vi "busy_wait.vi"(7 "caller":refnum<vi>, 8 "error in (no error)":errorcluster, 10 "configuration":T2={"dialog_text"="", "wait_s"=0.0, "inner_color"=16711680, "outer_color"=6618880, "event_registration"=refnum}, 11 "v1 in":refnum<class "v1.lvclass">) -> (0 "error out":errorcluster, 2 "dialog_selection":T1, 3 "v1 out":refnum<class "v1.lvclass">)   [LabVIEW 2015, in "lv-dialog.lvlib" / "v1.lvlib" / "v1.lvclass"]
doc: "The busy/wait api can be used to provide feedback when a process is going to take a long time, as implemented within the base api class, it doesn't have a lot of functional feedback aside from setting or unsetting busy. The configuration provides a time (in seconds), the dialog message as well as an event registration that can be used to indicate \"done\" from the outside.\n\nThis is implemented by the base api class (not the embedded) by using the \"Set Busy\" and \"Unset Busy\" VIs."
uses:
  v1.lvclass
  _controls/selection.ctl
  v1.lvlib
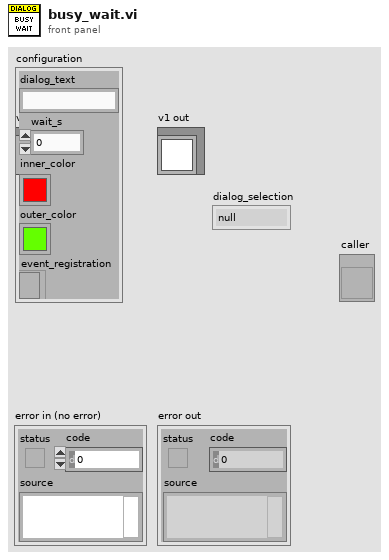
[diagram p1: front panel]
types:
  T1 = typedef "lv-dialog.lvlib/v1.lvlib/selection.ctl" = enum16{"null", "panel_closed", "button_1", "button_2", "button_3", "cancelled"}
  T2 = cluster{"dialog_text":string, "wait_s":dbl, "inner_color":u32, "outer_color":u32, "event_registration":refnum<event-registration>}
  T3 = cluster{"dialog_text":string, "boolean_text_1":string, "boolean_text_2":string}
  T4 = cluster{"dialog_text":string, "boolean_text_1":string}
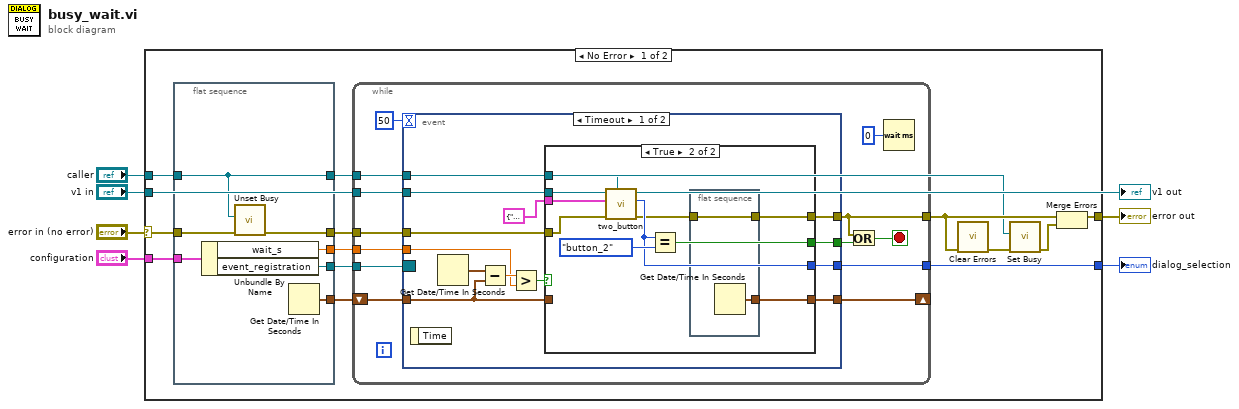
[diagram p0: block diagram]
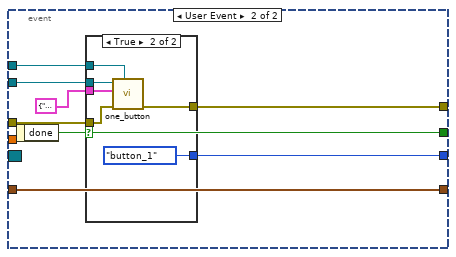
[diagram p3: hidden frame]
diagram:
  n1 = case shown="No Error" "error in (no error)" {
    selector: "error in (no error)" -> [w14 w83]
    tunnel: "configuration" -> [w20 _]
    tunnel: [w17 _] -> w5
    tunnel: "v1 in" -> [w16 _]
    tunnel: "caller" -> [w13 _]
    tunnel: [w9 w83] -> w1
    frame No Error {
      n2 = flat-sequence {
        tunnel: w20 -> [w27]
        tunnel: [w26] -> w19
        tunnel: [w25] -> w18
        tunnel: [w24] -> w15
        tunnel: w14 -> [w23]
        tunnel: w13 -> [w22]
        tunnel: [w22] -> w7
        tunnel: [w21] -> w12
        frame #0 {
          n3 = Unbundle By Name(w27) -> ("wait_s"=w24:dbl, "event_registration"=w25:refnum<event-registration>)
          n4 = call <vilib>:"Unset Busy.vi"("error in (no error)"=w23, "VI reference (current VI)"=w22) -> ("error out"=w21:errorcluster)  [unwired: 9 in]
          n5 = Get Date/Time In Seconds() -> (seconds since 1Jan1904=w26:timestamp)
        }
      }
      n6 = while {
        shift-right: [w36] -> _
        shift-left: w19 -> [w37]
        tunnel: w15 -> [w35]
        tunnel: w7 -> [w31]
        tunnel: [w30] -> w17
        tunnel: w18 -> [w29]
        tunnel: w16 -> [w28]
        tunnel: w12 -> [w40]
        tunnel: [w32] -> w8
        stop <- w33 stop-if-true
        n7 = event shown="[0] Timeout" {
          selector: w29 -> [_ _]
          dyn-events: _ -> [_ _]
          timeout: 50 -> [_ _]
          tunnel: w40 -> [w43 w75]
          tunnel: [w51 w74] -> w32
          tunnel: [w50 w70] -> w34
          tunnel: w37 -> [w46 w71]
          tunnel: [w45 w71] -> w36
          tunnel: w35 -> [w42 _]
          tunnel: w31 -> [w48 w73]
          tunnel: [w47 w69] -> w30
          tunnel: w28 -> [w41 w68]
          event Timeout {
            n8 = event-data() -> ()  [unwired: 1 in, 1 out]
            n9 = Get Date/Time In Seconds() -> (seconds since 1Jan1904=w53:timestamp)
            n10 = Subtract(x=w53, y=w46) -> (x-y=w52:dbl)
            n11 = Greater?(x=w52, y=w42) -> (0:w44:bool)
            n12 = case shown="True" w44 {
              tunnel: w43 -> [w55 w63]
              tunnel: [w55 w59] -> w51
              tunnel: [_ w64] -> w50
              tunnel: T3 {"dialog_text"="Waiting process has not completed.", "boolean_text_1"="Wait", "boolean_text_2"="Continue"} -> [_ w57]
              tunnel: w48 -> [_ w58]
              tunnel: [_ w62] -> w47
              tunnel: w46 -> [w54 _]
              tunnel: [w54 w61] -> w45
              tunnel: w41 -> [_ w56]
              frame False {
              }
              frame True {
                n13 = call-dynamic "two_button.vi"("callee"=w58, "error in (no error)"=w63, "configuration"=w57, "v1 in"=w56) -> ("error out"=w60:errorcluster, "dialog_selection"=w62:T1)  [unwired: 5 in, 1 out]
                n14 = Equal?(x=w62, y=selection."button_2" ("x")) -> (x = y?=w64:bool)
                n15 = flat-sequence {
                  tunnel: [w67] -> w61
                  tunnel: w60 -> [w66]
                  tunnel: [w66] -> w59
                  frame #0 {
                    n16 = Get Date/Time In Seconds() -> (seconds since 1Jan1904=w67:timestamp)
                  }
                }
              }
            }
          }
          event User Event {
            n17 = event-data() -> ("done"=w70:bool)  [unwired: 1 in]
            n18 = case shown="True" w70 {
              tunnel: w75 -> [w76 w82]
              tunnel: [w76 w81] -> w74
              tunnel: w73 -> [_ w80]
              tunnel: T4 {"dialog_text"="Process Complete", "boolean_text_1"="OK"} ("configuration") -> [_ w79]
              tunnel: [_ selection."button_1" ("dialog_selection")] -> w69
              tunnel: w68 -> [_ w77]
              frame False {
              }
              frame True {
                n19 = call-dynamic "one_button.vi"("callee"=w80, "error in (no error)"=w82, "configuration"=w79, "v1 in"=w77) -> ("error out"=w81:errorcluster)  [unwired: 5 in, 2 out]
              }
            }
          }
        }
        n20 = Or(x=w32, y=w34) -> (x .or. y?=w33:bool)
        n21 = Wait (ms)(milliseconds to wait=u32 0) -> ()  [unwired: 1 out]
      }
      n22 = call <vilib>:"Clear Errors.vi"("error in (no error)"=w8) -> ("error out"=w11:errorcluster)  [unwired: 5 in, 1 out]
      n23 = call <vilib>:"Set Busy.vi"("error in (no error)"=w11, "VI reference (current VI)"=w7) -> ("error out"=w10:errorcluster)  [unwired: 8 in, 1 out]
      n24 = Merge Errors(w8, w10) -> (w9:errorcluster)
    }
    frame Error {
    }
  }
  "error out" <- w1
  "dialog_selection" <- w5
  "v1 out" <- "v1 in"
